vi "Create Timing Channel Array.vi"(10 "timing channel ref":T1=18446744073709551615 format="%.0x", 11 "incoming channels (empty)":T1[](array[typedef]) format="%.0x") -> (2 "channel offset":i32, 3 "incoming channels out":T1[](array[typedef]) format="%.0x")   [LabVIEW 2020, in "AIM MIL-STD-1553 Engine.lvlib" / "Implementation.lvlib" / "Execution Unit Factory.lvclass"]
uses:
  Execution Unit Factory.lvclass
  <vilib>/NI VeriStand/Custom Device API/Custom Device Item Ref.ctl
  <vilib>/NI VeriStand/Custom Device API/Custom Device API.lvlib
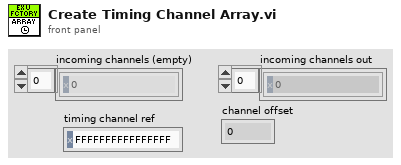
[diagram p1: front panel]
types:
  T1 = typedef "Custom Device API.lvlib/Custom Device Item Ref.ctl" = u64
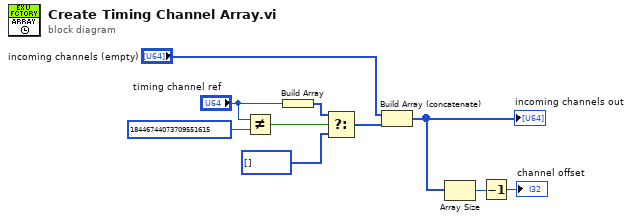
[diagram p0: block diagram]
diagram:
  n1 = Not Equal?(x="timing channel ref", y=T1 18446744073709551615) -> (x != y?=w9:bool)
  n2 = Build Array("timing channel ref") -> (w7:T1[])
  n3 = Select(t=w7, s=w9, f=T1[] []) -> (s? t:f=w3:T1[])
  n4 = Build Array (concatenate)("incoming channels (empty)", w3) -> (w1:T1[])
  "incoming channels out" <- w1
  n5 = Array Size(array=w1) -> (size(s)=w5:i32)
  n6 = Decrement(x=w5) -> (x-1=→"channel offset":i32)
